vi "z-scope.vi"() -> ()   [LabVIEW 2017]
uses:
  controls/boolean_info.ctl
  sysID_Z-axis-params.ctl
  <vilib>/rvi/Emulation/niFpgaGetClockAttributes.vi
  <vilib>/rvi/Emulation/niFpgaSctlEmulationGetInTimedLoop.vi
  <vilib>/rvi/Emulation/niFpgaEmulationReportErrorSimple.vi
  <vilib>/rvi/Emulation/niFpgaProcessEmulError.vi
  <vilib>/rvi/eio/common/nirviEmuTemplateMethod_errors.vi
  <vilib>/rvi/interface/RandomDataEmulation/niFpgaRandomDataHandleErrors.vi
  <vilib>/rvi/Emulation/niFpgaCriticalErrorInLSC.vi
  <vilib>/eio/EIONode/EIONode.xnode
  <vilib>/rvi/DataTransferAndStorage/Container/XNode/niFpgaContainer.xnode
  <vilib>/rvi/interface/RandomDataEmulation/nirviRandomDataFpgaReadWriteTemplate.vi
panel:
  in  "sysID_Z_axis_params":T1={"TOL"=0.3, "ramp-rate"=-5e-06, "z-u-max"=5.0, "offset"=0.0, "Ki"=0.001, "Z-error-threshold"=0.0, "Z-settled-samples\nthreshold "=0, "z_UP"=1.5, "zup-N"=5000} {"Z-error-threshold" format="%#_13g"; "ramp-rate" format="%#_4g"; "TOL" format="%#_13g"}
  out "iter":i32
  out "All Done":bool
  in  "TsTicks":u32=1600
  out "boolean \nindicators":T2
  out "z-u(k)":sgl
  in  "ABORT":bool
  # "- If collect all = fasle and collect move = false,\nwe only collect measurement data.\n- If collect all = false, and collect move = true,\nwe collect measurement and move data.\n- If collect all = true, we collect everything."
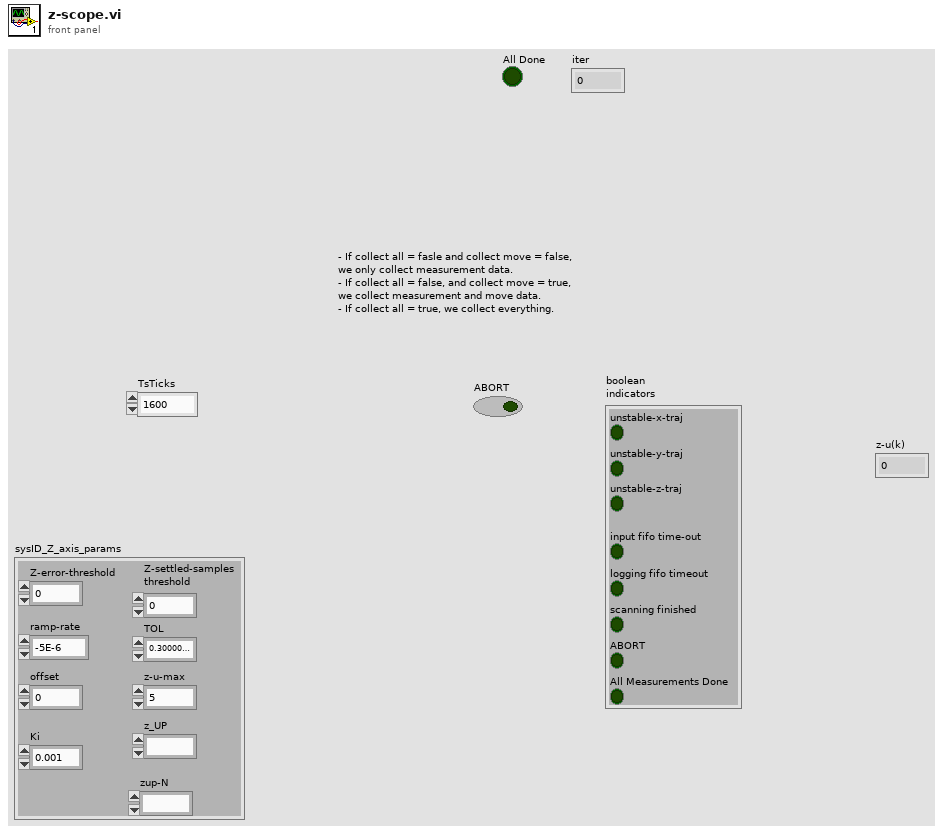
[diagram p1: front panel]
types:
  T1 = typedef "sysID_Z-axis-params.ctl" = cluster{"TOL":sgl, "ramp-rate":sgl, "z-u-max":sgl, "offset":sgl, "Ki":sgl, "Z-error-threshold":sgl, "Z-settled-samples\nthreshold ":i16, "z_UP":fxp<+/-,16,5>, "zup-N":i16}
  T2 = typedef "boolean_info.ctl" = cluster{"unstable-z-traj":bool, "input fifo time-out":bool, "logging fifo timeout":bool, "scanning finished":bool, "unstable-x-traj":bool, "unstable-y-traj":bool, "ABORT":bool, "All Measurements Done":bool}
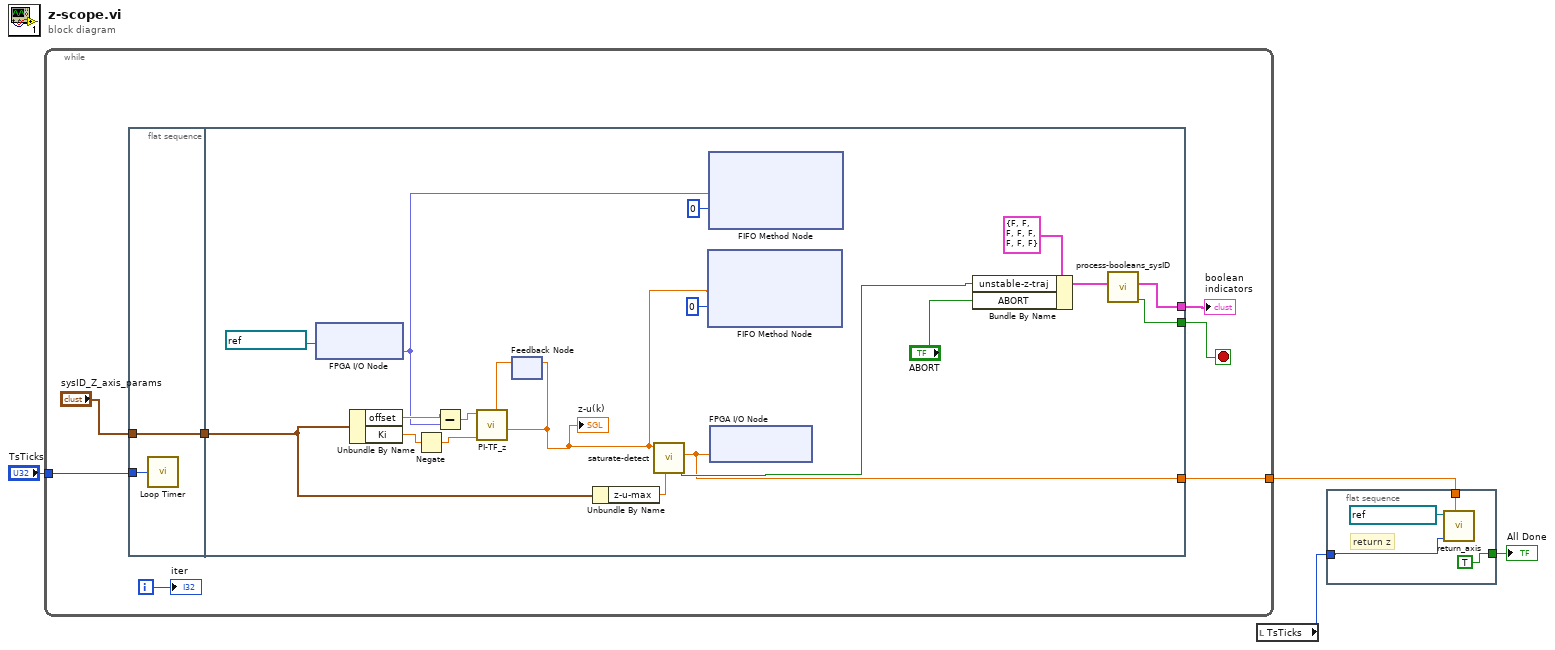
[diagram p0: block diagram]
diagram:
  n1 = while {
    tunnel: "TsTicks" -> [w10]
    tunnel: [w7] -> w3
    i -> [w6]
    stop <- w8 stop-if-true
    n2 = flat-sequence {
      tunnel: w10 -> [w12]
      tunnel: "sysID_Z_axis_params" -> [w13]
      tunnel: [w13] -> w11
      tunnel: [w26] -> w8
      tunnel: [w27] -> w9
      tunnel: [w29] -> w7
      tunnel: w11 -> [w22]
      frame #0 {
        n3 = call "Loop Timer"("Count(Ticks)"=w12) -> ()  [unwired: 1 out]
      }
      frame #1 {
        n4 = xnode "FPGA I/O Node"("FPGA I/O In"=refnum<k21> "Mod2/AI2" ("y - ADC")) -> ("I/O Item"=w17:fxp<+/-,24,5>)  [unwired: 1 out]
        n5 = Unbundle By Name(w22) -> ("offset"=w21:sgl, "Ki"=w20:sgl)
        n6 = Negate(x=w20) -> (-x=w19:sgl)
        n7 = Subtract(x=w21, y=w17) -> (x-y=w18:sgl)
        n8 = feedback #1() -> (w23:sgl)  [unwired: 1 in]
        n9 = call "PI-TF_z.vi"("u(k-1)"=w23, "Ki"=w19, "e(k)"=w18) -> ("u(k)"=w14:sgl)  [unwired: 8 in]
        "z-u(k)" <- w14
        n10 = feedback-in #1(w14) -> ()
        n11 = Unbundle By Name(w22) -> ("z-u-max"=w25:sgl)
        n12 = call "saturate-detect.vi"("bound"=w25, "x"=w14) -> ("saturated"=w32:bool, "sat(x)"=w29:sgl)  [unwired: 8 in]
        n13 = xnode ("FIFO Method Node")("Element"=w14, "Timeout"=0) -> ()  [unwired: 1 in, 2 out]
        n14 = xnode ("FIFO Method Node")("Element"=w17, "Timeout"=0) -> ()  [unwired: 1 in, 2 out]
        n15 = xnode "FPGA I/O Node"("Mod1/AO2"=w29) -> ()  [unwired: 1 in, 1 out]
        n16 = Bundle By Name(cluster=T2 {"unstable-z-traj"=FALSE, "input fifo time-out"=FALSE, "logging fifo timeout"=FALSE, "scanning finished"=FALSE, "unstable-x-traj"=FALSE, "unstable-y-traj"=FALSE, "ABORT"=FALSE, "All Measurements Done"=FALSE} ("boolean errors"), "unstable-z-traj"=w32, "ABORT"="ABORT") -> (w28:T2)
        n17 = call "process-booleans_sysID.vi"("boolean indicators 2"=w28) -> ("scaning finished"=w26:bool, "boolean indicators"=w27:T2)  [unwired: 9 in]
      }
    }
    "boolean \nindicators" <- w9
    "iter" <- w6
  }
  n18 = local read "TsTicks"() -> (w1:u32)
  n19 = flat-sequence {
    tunnel: w3 -> [w36]
    tunnel: [TRUE] -> w2
    tunnel: w1 -> [w33]
    frame #0 {
      # "return z"
      n20 = call "return_axis.vi"("u(0)"=w36, "TsTicks"=w33, "FPGA I/O In"=refnum<k21> "Mod1/AO2") -> ()  [unwired: 9 in]
    }
  }
  "All Done" <- w2
